vi "Write_Sub_Collection.vi"(8 "error in (no error)":errorcluster caption="entrée d'erreur (pas d'erreur)", 10 "fields":T1, 11 "Firebase PCBA en entrée":refnum<class "Firebase Packaging.lvclass">) -> (0 "error out":errorcluster caption="sortie d'erreur", 3 "Firebase PCBA en sortie":refnum<class "Firebase Packaging.lvclass">)   [LabVIEW 2020, in "Library Instrument & Equipement.lvlib" / "Library FireBase.lvlib" / "Firebase Packaging.lvclass"]
doc: "Create New document\nPlease initialise the following values\n - Name BDD\n - Document of test sequence\n - API Key"
uses:
  Firebase Packaging.lvclass
  Firebase Packaging.lvclass/Firebase Packaging.ctl
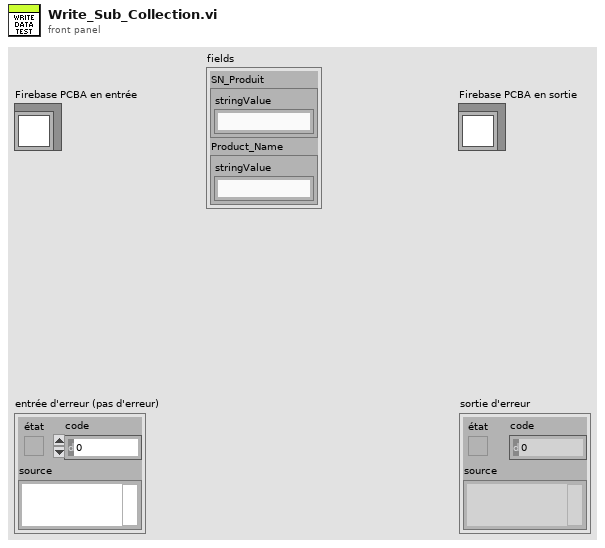
[diagram p1: front panel]
types:
  T1 = cluster{"SN_Produit":cluster{"stringValue":string}, "Product_Name":cluster{"stringValue":string}}
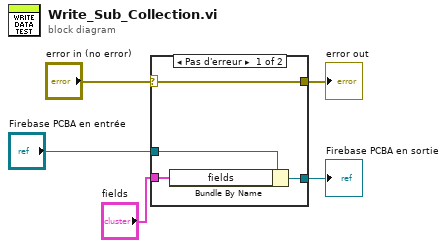
[diagram p0: block diagram]
diagram:
  n1 = case shown="Pas d'erreur" "error in (no error)" {
    selector: "error in (no error)" -> [w8 w11]
    tunnel: [w8 w11] -> w4
    tunnel: [w7 w10] -> w2
    tunnel: "Firebase PCBA en entrée" -> [w6 w10]
    tunnel: "fields" -> [w9 _]
    frame No Error {
      n2 = Bundle By Name(cluster=w6, "fields"=w9) -> (w7:refnum<class "Firebase Packaging.lvclass">)
    }
    frame Error {
    }
  }
  "error out" <- w4
  "Firebase PCBA en sortie" <- w2
